vi "Exit.vi"   [LabVIEW 2015]
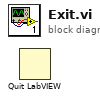
[diagram p0: block diagram]
diagram:
  n1 = Quit LabVIEW() -> ()  [unwired: 1 in]
